vi "TSCAN_SetData_Regs.vi"(8 "error in (no error)":errorcluster, 9 "CAN_Config_Regs":T1={"CAN_Sampling point"={"ASEG1"=0, "ASEG2"=0, "APrescaler"=0, "ASJW"=0}, "CAN configuration"={"HardwareType"=8, "Hardware Subtype"=enum."TC1016", "ABaudrateKbps"=250.0, "AListenOnly"=enum."Normal", "Int120Ohm"=enum."Enable", "EnableChannel"=enum."Enable", "AHwChannel"=0, "AAppChannel"=0, "AldHW"=0}} {"CAN configuration"."AAppChannel" items=["CHN1", "CHN2", "CHN3", "CHN4", "CHN5", "CHN6", "CHN7", "CHN8", "CHN9", "CHN10", "CHN11", "CHN12", "CHN13", "CHN14", "CHN15", "CHN16", "CHN17", "CHN18", "CHN19", "CHN20", "CHN21", "CHN22", "CHN23", "CHN24", "CHN25", "CHN26", "CHN27", "CHN28", "CHN29", "CHN30", "CHN31", "CHN32"]; "CAN configuration"."AHwChannel" items=["CHN1", "CHN2", "CHN3", "CHN4", "CHN5", "CHN6", "CHN7", "CHN8", "CHN9", "CHN10", "CHN11", "CHN12", "CHN13", "CHN14", "CHN15", "CHN16", "CHN17", "CHN18", "CHN19", "CHN20", "CHN21", "CHN22", "CHN23", "CHN24", "CHN25", "CHN26", "CHN27", "CHN28", "CHN29", "CHN30", "CHN31", "CHN32"]; "CAN configuration"."HardwareType" items=["BUS_UNKNOWN_TYPE", "TS_TCP_DEVICE", "XL_USB_DEVICE", "TS_USB_DEVICE", "PEAK_USB_DEVICE", "KVASER_USB_DEVICE", "ZLG_USB_DEVICE", "ICS_USB_DEVICE", "TS_TC1005_DEVICE", "CANABLE_USB_DEVICE", "TS_WIRELESS_OBD", "TS_USB_DEVICE_EX", "IXXAT_USB_DEVICE", "TS_ETH_IF_DEVICE", "TS_USB_IF_DEVICE", "BUS_DEV_TYPE_COUNT"]}, 10 "FAPppName":string, 11 "Path":path) -> (0 "error out":errorcluster, 3 "Path output":path, 4 "Config_retuen":i32, 6 "maping_retuen":i32)   [LabVIEW 2014]
doc: "tsapp_set_mapping_verbose ：\nFunction Introduction ：\nBefore using hardware devices, map the channels (CAN/CANFD/LIN) for the application program\n(i.e. binding) specifies the designated channel of the CAN device. This operation can also be performed on\nThe device management interface of TSMaster is completed, and this part of the operation is not required in the code.\nRegarding the channel mapping function, there are still unclear areas. Please refer to the document: TsMasterApi HardwareMap.pdf\nCall location ：\nCall this function to complete the hardware binding before the application connects to the CAN tool.\ninput parameter \nAppName: Application Name: The name of the application bound to this Map, which should be consistent with the name in initialized lib_tsmaster\nagreement\nAAppChannelType: Channel type: including APP_CAN, APP_LIN AAppChannel: Channel number of the application: This is the channel number used by the upper level program\nAHardwareName: Hardware name: such as TOSUN, Vector, etc., can also be left blank, mainly for the convenience of users to view\nAHardwareType: Hardware type: According to TLIBBusToolDeviceType, it includes all mainstream CANs currently on the market\nCard hardware Among them, the definition of tool enumeration types is as follows:\npublic enum TLIBBusToolDeviceType : int {\nBUS_UNKNOWN_TYPE = 0, TS_TCP_DEVICE = 1, XL_USB_DEVICE = 2, TS_USB_DEVICE = 3, PEAK_USB_DEVICE = 4, KVASER_USB_DEVICE = 5, ZLG_USB_DEVICE = 6, ICS_USB_DEVICE = 7, TS_TC1005_DEVICE = 8\n};\nAHardwareSubType: The sub devices under this device type, such as TS-USB-Device on the same star, are included below TC1001, TL1002, TC1011 and other series of products\nAHardwareIndex: Supports inserting multiple identical hardware devices simultaneously, such as inserting two TC1001 devices at the same time. This is used to select\nIs it the channel of device 1 or device 2\nAHardwareChannel: The channel for hardware devices, for example, TC1005 has 5 hardware channels, and this parameter is used to select the appropriate one\nCorresponding hardware channels\nAEnable Mapping: Is this mapping enabled? If set to false, the channel cannot be used。\nReturn value ：\n==0: Execution successful\nOther: Query error code\n\n\ntsapp_configure_baudrate_can ：\nFunction Introduction ：\nSet parameters such as baud rate for CAN channel\nCall location ：\nBefore connecting hardware devices, set the parameters of the channel first\ninput parameter ：\nAIdxChn: Application Channel Number\nABaud rate Kbps: baud rate (kbps)\nAListenOnly: Whether to only listen mode, if enabled, can only receive data\nAInstallTermResistor120Ohm: Can only internal terminal resistors of the device be used\nReturn value ：\n==0: Connection successful\nOther: Check for error codesS"
uses:
  Utilities/Typedef/Hardware_Subtype.ctl
  Typedef/TSCAN_CAN_Configuration.ctl
  Typedef/TSCAN_CAN_Configuration_Regs.ctl
  All_Control/Typedef/Hardware Type.ctl
panel:
  # "Use N CAN channels and set N CAN channels"
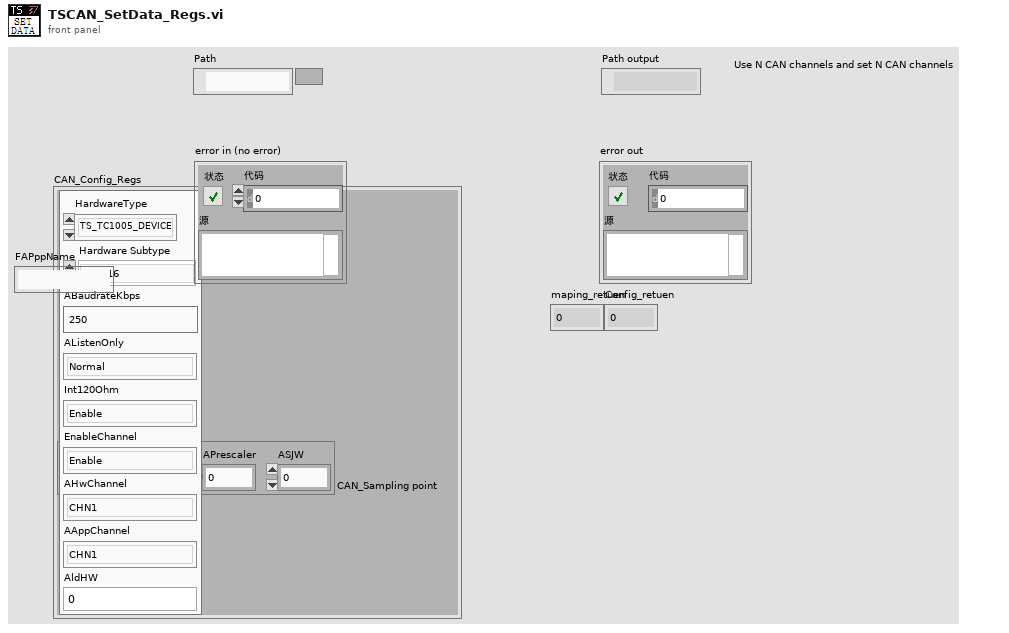
[diagram p1: front panel]
types:
  T1 = typedef "TSCAN_CAN_Configuration_Regs.ctl" = cluster{"CAN_Sampling point":cluster{"ASEG1":i32, "ASEG2":i32, "APrescaler":i32, "ASJW":i32}, "CAN configuration":T2}
  T2 = typedef "TSCAN_CAN_Configuration.ctl" = cluster{"HardwareType":T3, "Hardware Subtype":T4, "ABaudrateKbps":sgl, "AListenOnly":enum16{"Normal", "ListenOnly"}, "Int120Ohm":enum16{"Disable", "Enable"}, "EnableChannel":enum16{"Disable", "Enable"}, "AHwChannel":i32, "AAppChannel":i32, "AldHW":i32}
  T3 = typedef "Hardware Type.ctl" = i32
  T4 = typedef "Hardware_Subtype.ctl" = enum16{"TS_UNKNOWN_DEVICE", "TSCAN_PRO", "TSCAN_Lite1", "TC1001", "TL1001", "TC1011", "TM5011", "TC1002", "TC1014", "TSCANFD2517", "TC1026", "TC1016", "TC1012", "TC1013", "TLog1002", "TC1034", "TC1018", "GW2116", "TC2115", "MP1013", "TC1113", "TC1114", "TP1013", "TC1017", "TP1018", "TF10XX", "TL1004_FD_4_LIN_2", "TE1051", "TP1051", "TP1034", "TTS9015", "TP1026", "TTS1026", "TTS1034", "TTS1018", "TL1011", "TTS1015_LiAuto", "TTS1013_LiAuto", "TTS1016Pro", "TC1054Pro", "TC1054", "TLog1038", "TO1013", "TC1034Pro", "TC1018Pro", "TC1038Pro", "TS_DEV_END"}
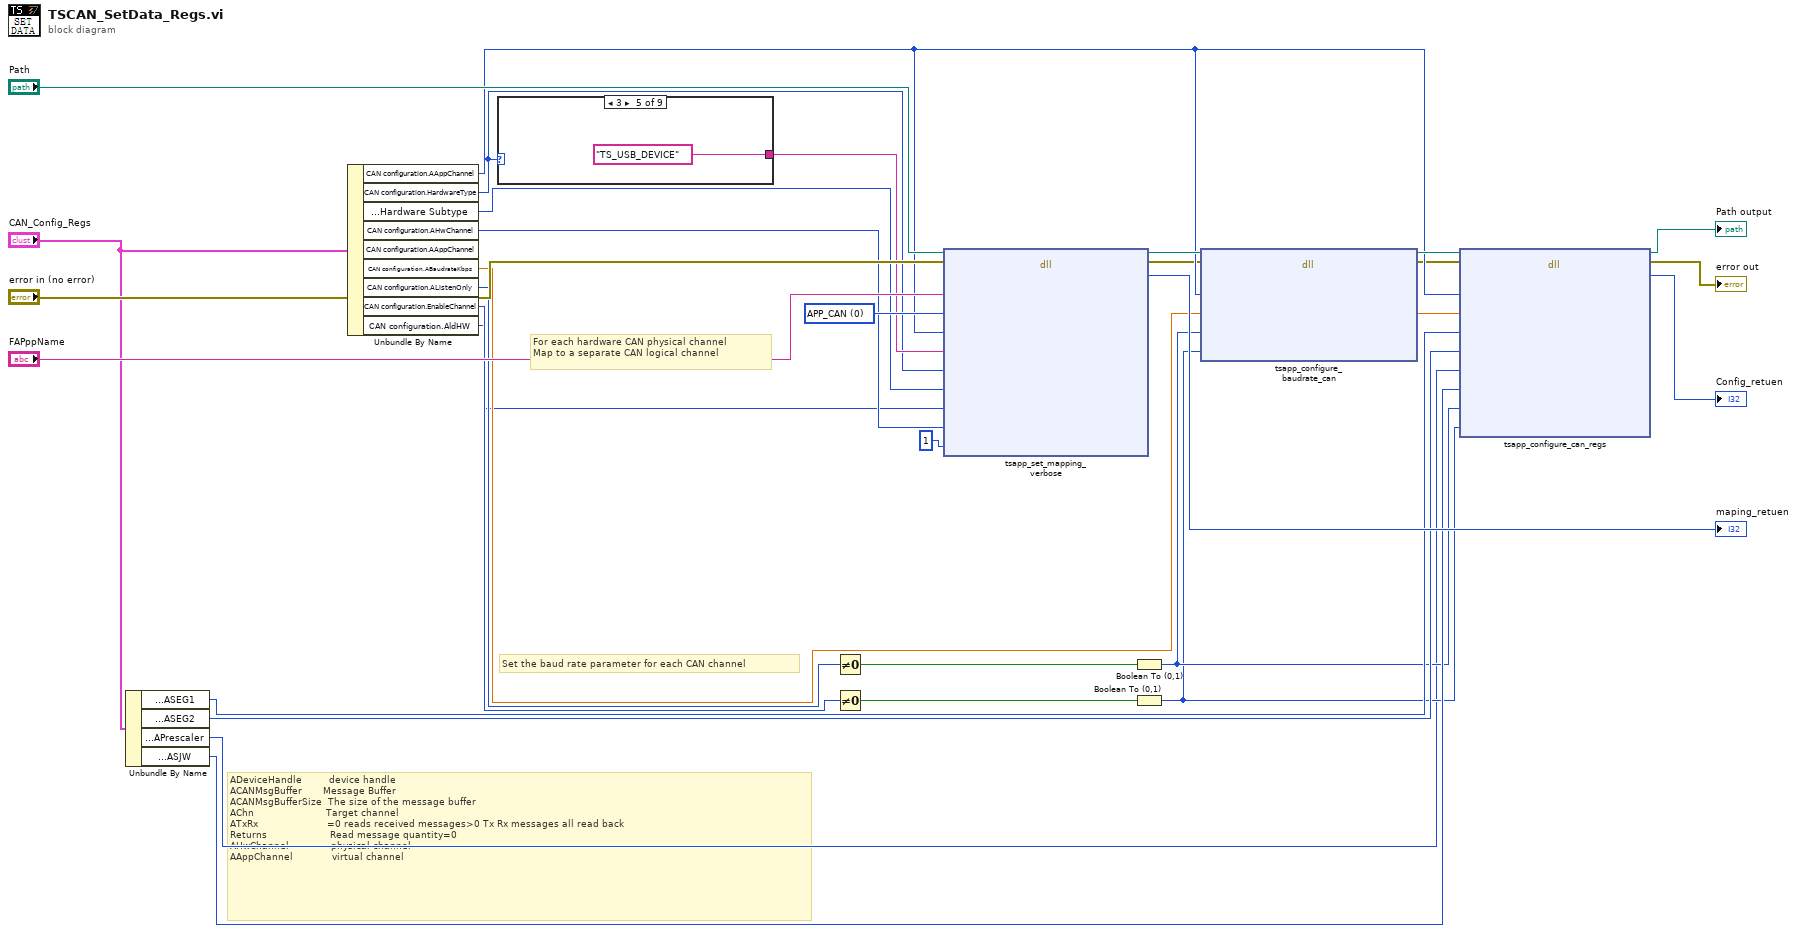
[diagram p0: block diagram]
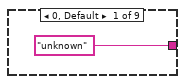
[diagram p2: hidden frame]
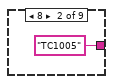
[diagram p3: hidden frame]
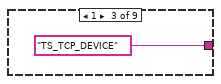
[diagram p4: hidden frame]
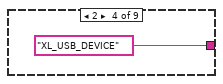
[diagram p5: hidden frame]
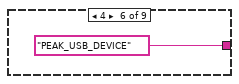
[diagram p6: hidden frame]
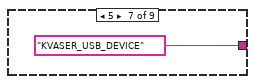
[diagram p7: hidden frame]
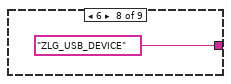
[diagram p8: hidden frame]
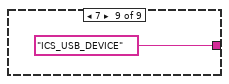
[diagram p9: hidden frame]
diagram:
  w29 = 0 items=["APP_CAN", "APP_LIN"] ("AAppChannelType")
  # "For each hardware CAN physical channel\nMap to a separate CAN logical channel"
  # "ADeviceHandle         device handle\nACANMsgBuffer       Message Buffer\nACANMsgBufferSize  The size of the message buffer\nAChn                        Target channel\nATxRx                       =0 reads received messages>0 Tx Rx messages all read back\nReturns                     Read message quantity=0\nAHwChannel              physical channel\nAAppChannel             virtual channel"
  # "Set the baud rate parameter for each CAN channel"
  n1 = Unbundle By Name("CAN_Config_Regs") -> ("CAN_Sampling point.ASEG1"=w15:i32, "CAN_Sampling point.ASEG2"=w14:i32, "CAN_Sampling point.APrescaler"=w1:i32, "CAN_Sampling point.ASJW"=w13:i32)
  n2 = Unbundle By Name("CAN_Config_Regs") -> ("CAN configuration.AAppChannel"=w9:i32, "CAN configuration.HardwareType"=w27:T3, "CAN configuration.Hardware Subtype"=w26:T4, "CAN configuration.AHwChannel"=w25:i32, "CAN configuration.ABaudrateKbps"=w6:sgl, "CAN configuration.AListenOnly"=w21:enum16{"Normal", "ListenOnly"}, "CAN configuration.EnableChannel"=w20:enum16{"Disable", "Enable"}, "CAN configuration.AldHW"=w2:i32)  [unwired: 1 out]
  n3 = case shown="3" w27 {
    tunnel: ["unknown" ("AHardwareName") "TC1005" ("AHardwareName") "TS_TCP_DEVICE" ("AHardwareName") "XL_USB_DEVICE" ("AHardwareName") "TS_USB_DEVICE" ("AHardwareName") "PEAK_USB_DEVICE" ("AHardwareName") "KVASER_USB_DEVICE" ("AHardwareName") "ZLG_USB_DEVICE" ("AHardwareName") "ICS_USB_DEVICE" ("AHardwareName")] -> w28
    frame 0, Default {
    }
    frame 8 {
    }
    frame 1 {
    }
    frame 2 {
    }
    frame 3 {
    }
    frame 4 {
    }
    frame 5 {
    }
    frame 6 {
    }
    frame 7 {
    }
  }
  n4 = Not Equal To 0?(x=w21) -> (x != 0?=w23:bool)
  n5 = Not Equal To 0?(x=w20) -> (x != 0?=w22:bool)
  n6 = dll-call lib="PTH2Habs CUsers\nAdministratorDesktopTS_Can通讯PathTSMaster.dll" fn="tsapp_set_mapping_verbose"(path in="Path", error in="error in (no error)", "FAPppName"="FAPppName", "AChnType"=w29, "FAppChannelIndex"=w9, "AHWDeviceName"=w28, "AHWDeviceType"=w27, "AHWDeviceSubType"=w26, "AldHW"=w2, "AldHWChn"=w25, "FMappingDisabled"=u32 1) -> (path out=w11:path, error out=w8:errorcluster, "tsapp_set_mapping_verbose"=→"maping_retuen":i32)  [unwired: 10 in]
  n7 = Boolean To (0,1)(Boolean=w23) -> (0, 1=w4:i16)
  n8 = Boolean To (0,1)(Boolean=w22) -> (0, 1=w3:i16)
  n9 = dll-call lib="PTH2Habs CUsers\nAdministratorDesktopTS_Can通讯PathTSMaster.dll" fn="tsapp_configure_baudrate_can"(path in=w11, error in=w8, "ALdxChn"=w9, "ABaudrateKbps"=w6, "AlistenOnly"=w4, "AlnstallTermResistor120Ohm"=w3) -> (path out=w10:path, error out=w7:errorcluster, "ABaudrateKbps"=w5:sgl)  [unwired: 5 in]
  n10 = dll-call lib="C:/Users/XYY/Desktop/LabView Demo/TSCAN_LB2018_V1.3_20220301/Config/TSMaster.dll" fn="tsapp_configure_can_regs"(path in=w10, error in=w7, "AIdxChn"=w9, "ABaudrateKbps"=w5, "ASEG1"=w15, "ASEG2"=w14, "APrescaler"=w1, "ASJW"=w13, "AOnlyListen"=w4, "A120OhmConnected"=w3) -> (path out=→"Path output":path, error out=→"error out":errorcluster, "返回类型"=→"Config_retuen":i32)  [unwired: 9 in]
